vi "Create and Read Recordset.vi"(6 "Max Rows to Fetch (-1 = all)":i32=-1, 8 "error in (no error)":errorcluster, 9 "Recordset Parameters":cluster{"CursorType":T1, "LockType":T2}={"CursorType"=0, "LockType"=1} {"LockType" items=["adLockUnspecified"=-1, "adLockReadOnly"=1, "adLockPessimistic"=2, "adLockOptimistic"=3, "adLockBatchOptimistic"=4]; "CursorType" items=["adOpenUnspecified"=-1, "adOpenForwardOnly"=0, "adOpenKeyset"=1, "adOpenDynamic"=2, "adOpenStatic"=3]}, 10 "Source":string, 11 "Connection In":refnum<k7>) -> (0 "error out":errorcluster, 1 "Rows Returned":i32, 2 "Selection Data":string[][](table), 3 "Connection Out":refnum<k7>, 4 "Field Names Fetched":string[](array[string]))   [LabVIEW 2022 SP3, in "hse-db-ado.lvlib" / "ADO-DB-Driver.lvlib"]
doc: "Create and read a recordset\n\n____\nHAMPEL SOFTWARE ENGINEERING v1.4.0 (2023-12-19 09:52)"
uses:
  ADO-DB-Driver.lvlib
  _typedefs/CursorType.ctl
  _typedefs/LockType.ctl
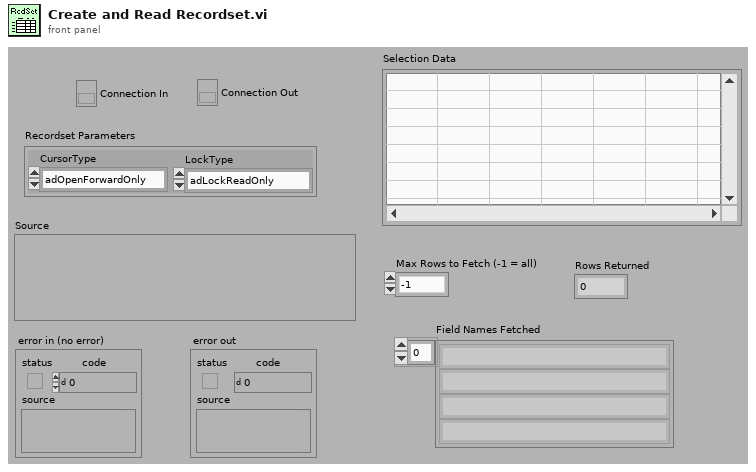
[diagram p1: front panel]
types:
  T1 = typedef "hse-db-ado.lvlib/ADO-DB-Driver.lvlib/CursorType.ctl" = i32
  T2 = typedef "hse-db-ado.lvlib/ADO-DB-Driver.lvlib/LockType.ctl" = i32
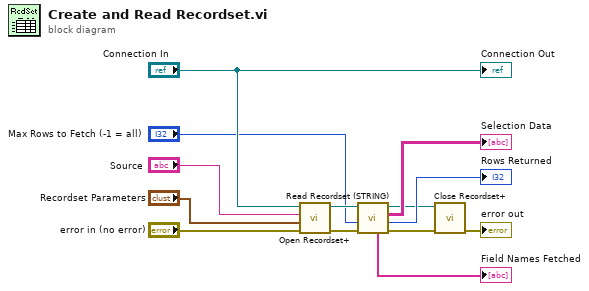
[diagram p0: block diagram]
diagram:
  n1 = call "Open Recordset+.vi"("error in (no error)"="error in (no error)", "Recordset Parameters"="Recordset Parameters", "Source"="Source", "Connection"="Connection In") -> ("error out"=w13:errorcluster, "Recordset"=w12:refnum<k7>)  [unwired: 6 in]
  n2 = call "Read Recordset (STRING).vi"("error in (no error)"=w13, "Max Rows to Fetch (-1 = all)"="Max Rows to Fetch (-1 = all)", "Recordset In"=w12) -> ("error out"=w11:errorcluster, "Rows Returned"=→"Rows Returned":i32, "Data out"=→"Selection Data":string[][], "Recordset Out"=w7:refnum<k7>, "Field Names"=→"Field Names Fetched":string[])  [unwired: 4 in]
  n3 = call "Close Recordset+.vi"("error in"=w11, "Recordset"=w7) -> ("error out"=→"error out":errorcluster)  [unwired: 9 in]
  "Connection Out" <- "Connection In"
